vi "PCA ComputeRetainedVariance.vi"(4 "retainedVariance":dbl=1.0, 6 "Flags":T1, 8 "error in (no error)":errorcluster, 9 "Mean":dbl[][](array[numeric]), 10 "Data":dbl[][](array[numeric]), 11 "PCA in":refnum<class "PCA.lvclass">) -> (0 "error out":errorcluster, 3 "PCA out":refnum<class "PCA.lvclass">)   [LabVIEW 2020, in "OpenLvVision_OpenCv.lvlib" / "PCA.lvclass"]
doc: "Performs PCA of the supplied dataset. It is safe to reuse the same PCA structure for multiple datasets. That is, if the structure has been previously used with another dataset, the existing internal data is reclaimed and the new eigenvalues, eigenvectors and mean are allocated and computed."
uses:
  PCA.lvclass
  C:/Users/lukas/Downloads/OpenLvVision_OpenCv/SourceCode/LabView/OpenLvVision_OpenCv/_LvHelpers/EdvrObject/EdvrObject.lvclass
  TypeDef/Flags.ctl
  _LvHelpers/EdvrObject/EdvrObject.lvclass/EdvrObject.ctl
  _LvHelpers/MatHandling/RegisterMat/RegisterMat_Array2D-DBL.vi
  OpenLvVision_OpenCv.lvlib
  _LvHelpers/EdvrObject/EdvrObject.lvclass
  Dlls/OlvOpenCvWrapper.dll
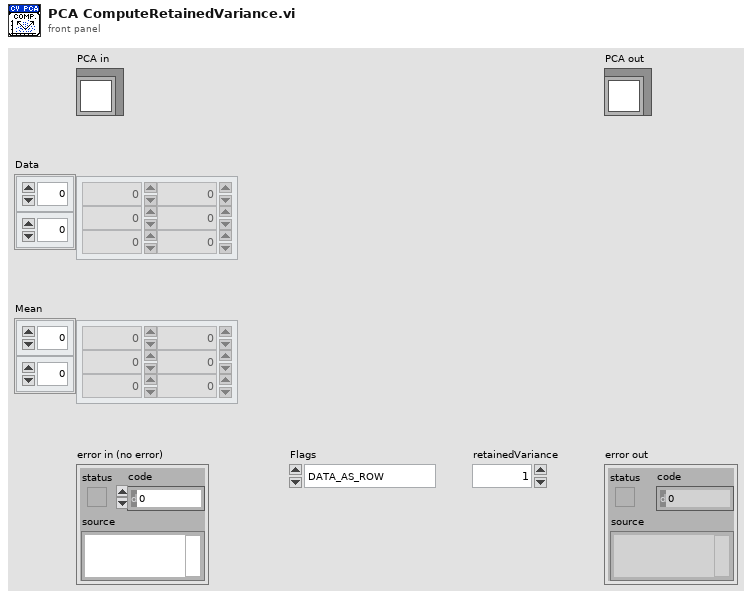
[diagram p1: front panel]
types:
  T1 = typedef "OpenLvVision_OpenCv.lvlib/PCA.lvclass/Flags.ctl" = enum32{"DATA_AS_ROW", "DATA_AS_COL", "USE_AVG"}
  T2 = typedef "OpenLvVision_OpenCv.lvlib/MatInfo.ctl" = cluster{"Datatype":T3, "Height":i32, "Width":i32, "Channels":i32, "LineWidth":i32, "Null":u8}
  T3 = typedef "OpenLvVision_OpenCv.lvlib/LvDatatype.ctl" = enum32{"Undefined", "U8", "I8", "U16", "I16", "U32_Color", "I32", "U64_Color", "I64", "SGL", "DBL", "Complex SGL", "Complex DBL", "Array 1D U8", "Array 1D I8", "Array 1D U16", "Array 1D I16", "Array 1D U32_Color", "Array 1D I32", "Array 1D U64_Color", "Array 1D I64", "Array 1D SGL", "Array 1D DBL", "Array 1D Complex SGL", "Array 1D Complex DBL", "Array 2D U8", "Array 2D I8", "Array 2D U16", "Array 2D I16", "Array 2D U32", "Array 2D U32_Color", "Array 2D I32", "Array 2D U64", "Array 2D U64_Color", "Array 2D I64", "Array 2D SGL", "Array 2D DBL", "Array 2D Complex SGL", "Array 2D Complex DBL", "Image Mono U8", "Image Mono U16", "Image Mono I16", "Image Mono SGL", "Image Color U32", "Image Color U64", "ImageComplex Sgl", "Array1d_2dPointI32", "Array1d_2dPointSGL", "Array1d_2dPointDBL", "Array1d_3dPointI32", "Array1d_3dPointSGL", "Array1d_3dPointDBL", "Array1d_4dPointI32", "Array1d_4dPointSGL", "Array1d_4dPointDBL"}
  T4 = typedef "OpenLvVision_OpenCv.lvlib/EdvrObject.lvclass/Edvr.ctl" = refnum<data-value>
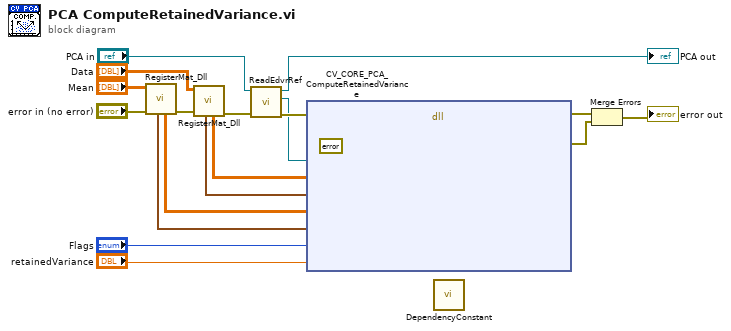
[diagram p0: block diagram]
diagram:
  n1 = call-poly "RegisterMat_Dll.vi"("error in"="error in (no error)", "Array in"="Mean") -> ("error out"=w9:errorcluster, "AdressOrData"=w8:dbl[][], "Mat"=w7:T2)  [unwired: 6 in, 1 out]
  n2 = call-poly "RegisterMat_Dll.vi"("error in"=w9, "Array in"="Data") -> ("error out"=w4:errorcluster, "AdressOrData"=w6:dbl[][], "Mat"=w5:T2)  [unwired: 6 in, 1 out]
  n3 = call "ReadEdvrRef.vi"("error in (no error)"=w4, "EdvrObject in"="PCA in") -> ("error out"=w3:errorcluster, "Edvr"=w2:T4, "EdvrObject out"=→"PCA out":refnum<class "PCA.lvclass">)  [unwired: 7 in]
  n4 = dll-call lib="C:/Users/lukas/Downloads/OpenLvVision_OpenCv/SourceCode/LabView/OpenLvVision_OpenCv/Dlls/OlvOpenCvWrapper.dll" fn="CV_CORE_PCA_ComputeRetainedVariance"(error in=w3, "Error"=errorcluster {"status"=FALSE, "code"=0, "source"=""} ("error out"), "edvrRef"=w2, "addressData"=w6, "matInfoData"=w5, "addressMean"=w8, "matInfoMean"=w7, "flags"="Flags", "RetainedVariance"="retainedVariance") -> (error out=w11:errorcluster, "Error"=w10:errorcluster)  [unwired: 10 in, 1 out]
  n5 = call "DependencyConstant.vi"() -> ()  [unwired: 12 in]
  n6 = Merge Errors(w11, w10) -> (→"error out":errorcluster)
